vi "fgv_f9p-latlong.vi"(7 "cmd":enum16{"write", "read"}(ring), 8 "error in":errorcluster, 10 "agv curr utm in":cluster{dbl, dbl}={530126.7583503594, 175270.68061157822} {"?" format="%.2f"; "?" format="%.2f"}, 11 "agv latlong":cluster{dbl, dbl}={530126.7583503594, 175270.68061157822} {"?" format="%.2f"; "?" format="%.2f"}) -> (0 "error out":errorcluster, 2 "utm out":cluster{dbl, dbl}={530126.7583503594, 175270.68061157822} {"?" format="%.2f"; "?" format="%.2f"}, 3 "latlong out":cluster{dbl, dbl}={530126.7583503594, 175270.68061157822} {"?" format="%.8f"; "?" format="%.8f"})   [LabVIEW 2019]
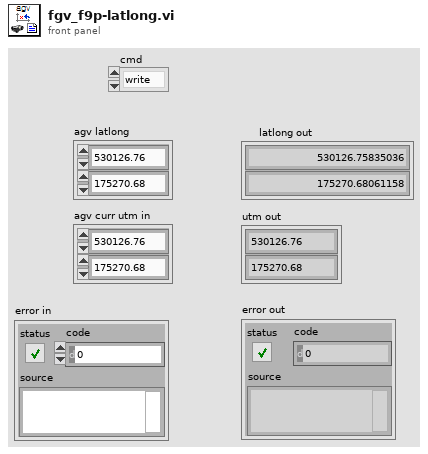
[diagram p1: front panel]
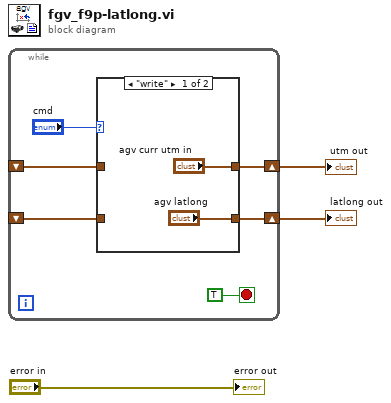
[diagram p0: block diagram]
diagram:
  n1 = while {
    shift-right: [w8] -> w3
    shift-left: _ -> [w7]
    shift-right: [w5] -> w1
    shift-left: _ -> [w4]
    stop <- TRUE stop-if-true
    n2 = case shown="\"write\"" "cmd" {
      tunnel: ["agv curr utm in" w13] -> w8
      tunnel: w7 -> [_ w13]
      tunnel: ["agv latlong" w12] -> w5
      tunnel: w4 -> [_ w12]
      frame "write" {
      }
      frame "read", Default {
      }
    }
  }
  "utm out" <- w3
  "latlong out" <- w1
  "error out" <- "error in"
